vi "sublijnvolgen.vi"(11 "Array":i32[](array[numeric])) -> (3 "Numeric 2":i32)   [LabVIEW 2019]
uses:
  <vilib>/myRIO/Instrument Drivers/Onboard IO/AO/typedefs/AO Reference.ctl
  <vilib>/myRIO/Common/Instrument Driver Framework/Utilities/typedefs/myRIO Generic Hardware Reference.ctl
  <vilib>/myRIO/Common/Instrument Driver Framework/Utilities/typedefs/Hardware Version Enum.ctl
  <vilib>/myRIO/Common/Instrument Driver Framework/Utilities/typedefs/myRIO v1.0 Reference.ctl
  <vilib>/myRIO/Common/Instrument Driver Framework/Utilities/typedefs/Generic FPGA Reference.ctl
  <vilib>/myRIO/Common/Instrument Driver Framework/myRIO v1.0/AO/typedefs/AO Channels List.ctl
  <vilib>/myRIO/Common/Instrument Driver Framework/myRIO v1.0/AO/typedefs/AO Channels Enum.ctl
  <vilib>/myRIO/Common/Instrument Driver Framework/Utilities/typedefs/Analog Scaling Constants List.ctl
  <vilib>/myRIO/Common/Instrument Driver Framework/Utilities/typedefs/Analog Scaling Constants.ctl
  <vilib>/userDefined/High Color/nirio_resource_hc.ctl
  <vilib>/myRIO/Common/Instrument Driver Framework/Utilities/vis/Is FPGA Ref Available.vi
  <vilib>/myRIO/Common/Instrument Driver Framework/myRIO v1.0/AO/vis/myRIO v1.1 Open AO.vi
  <vilib>/myRIO/Instrument Drivers/Onboard IO/AO/vis/Write.vi
  <vilib>/myRIO/Common/Instrument Driver Framework/Utilities/vis/Validate Channels.vi
  <vilib>/myRIO/Common/Instrument Driver Framework/myRIO v1.0/AO/vis/myRIO v1.0 Reserve AO.vi
  <vilib>/myRIO/Common/Instrument Driver Framework/myRIO v1.0/AO/vis/myRIO v1.0 Build MUX Configuration AO.vi
  <vilib>/myRIO/Common/Instrument Driver Framework/myRIO v1.0/Resource Manager/vis/myRIO v1.0 Reserve Channel List.vi
  <vilib>/myRIO/Common/Instrument Driver Framework/myRIO v1.0/Resource Manager/vis/myRIO v1.0 Reserve Channel.vi
  <vilib>/myRIO/Common/Instrument Driver Framework/myRIO v1.0/Resource Manager/vis/myRIO v1.0 Unreserve Channel.vi
  <vilib>/myRIO/Common/Instrument Driver Framework/myRIO v1.0/Resource Manager/vis/myRIO v1.0 Build Mutex Name.vi
  <vilib>/Utility/VariantDataType/GetNumericInfo.vi
  <vilib>/Utility/error.llb/Error Cluster From Error Code.vi
  <vilib>/myRIO/Common/Instrument Driver Framework/myRIO v1.0/myRIO v1.1 Open.vi
  <vilib>/myRIO/Common/Instrument Driver Framework/myRIO v1.0/AO/vis/myRIO v1.0 Get Scaling Constants AO.vi
  <vilib>/myRIO/Common/Instrument Driver Framework/Utilities/vis/IO Manager.vi
  <vilib>/myRIO/Common/Instrument Driver Framework/Utilities/vis/Configuration Manager.vi
  <vilib>/myRIO/Common/Instrument Driver Framework/myRIO v1.0/myRIO v1.0 Close.vi
  <vilib>/myRIO/Common/Instrument Driver Framework/myRIO v1.0/AO/vis/myRIO v1.0 Write AO.vi
  <vilib>/myRIO/Express VI/Onboard IO/AO/AO Express VI.xnode
  <vilib>/myRIO/Instrument Drivers/Onboard IO/AO/vis/myRIO AO Open.xnode
  <vilib>/myRIO/Instrument Drivers/Onboard IO/AO/AO.lvlib
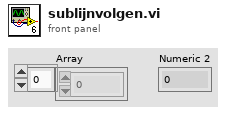
[diagram p1: front panel]
types:
  T1 = typedef "AO.lvlib/AO Reference.ctl" = cluster{"myRIO Reference":T2, "AO Channel List":T6, "AO Scaling Constant List":T8}
  T2 = typedef "myRIO Generic Hardware Reference.ctl" = cluster{"myRIO Model":T3, "myRIO Hardware Reference":T4}
  T3 = typedef "Hardware Version Enum.ctl" = enum16{"Unknown", "myRIO-1900", "myRIO-1950", "roboRIO", "NI ELVIS RIO CM", "ELVIS III"}
  T4 = typedef "myRIO v1.0 Reference.ctl" = cluster{"Generic FPGA Reference":T5, "Allow multiple opens":bool}
  T5 = typedef "Generic FPGA Reference.ctl" = refnum<k20>
  T6 = typedef "AO Channels List.ctl" = T7[]
  T7 = typedef "AO Channels Enum.ctl" = enum16{"Not Connected", "AudioOut/Left", "AudioOut/Right", "C/AO0", "C/AO1", "A/AO0", "A/AO1", "B/AO0", "B/AO1"}
  T8 = typedef "Analog Scaling Constants List.ctl" = T9[]
  T9 = typedef "Analog Scaling Constants.ctl" = cluster{"LSB Weight (Volts)":dbl, "Offset (Volts)":dbl, "Signed?":bool}
  T10 = typedef "nirio_resource_hc.ctl" = tag
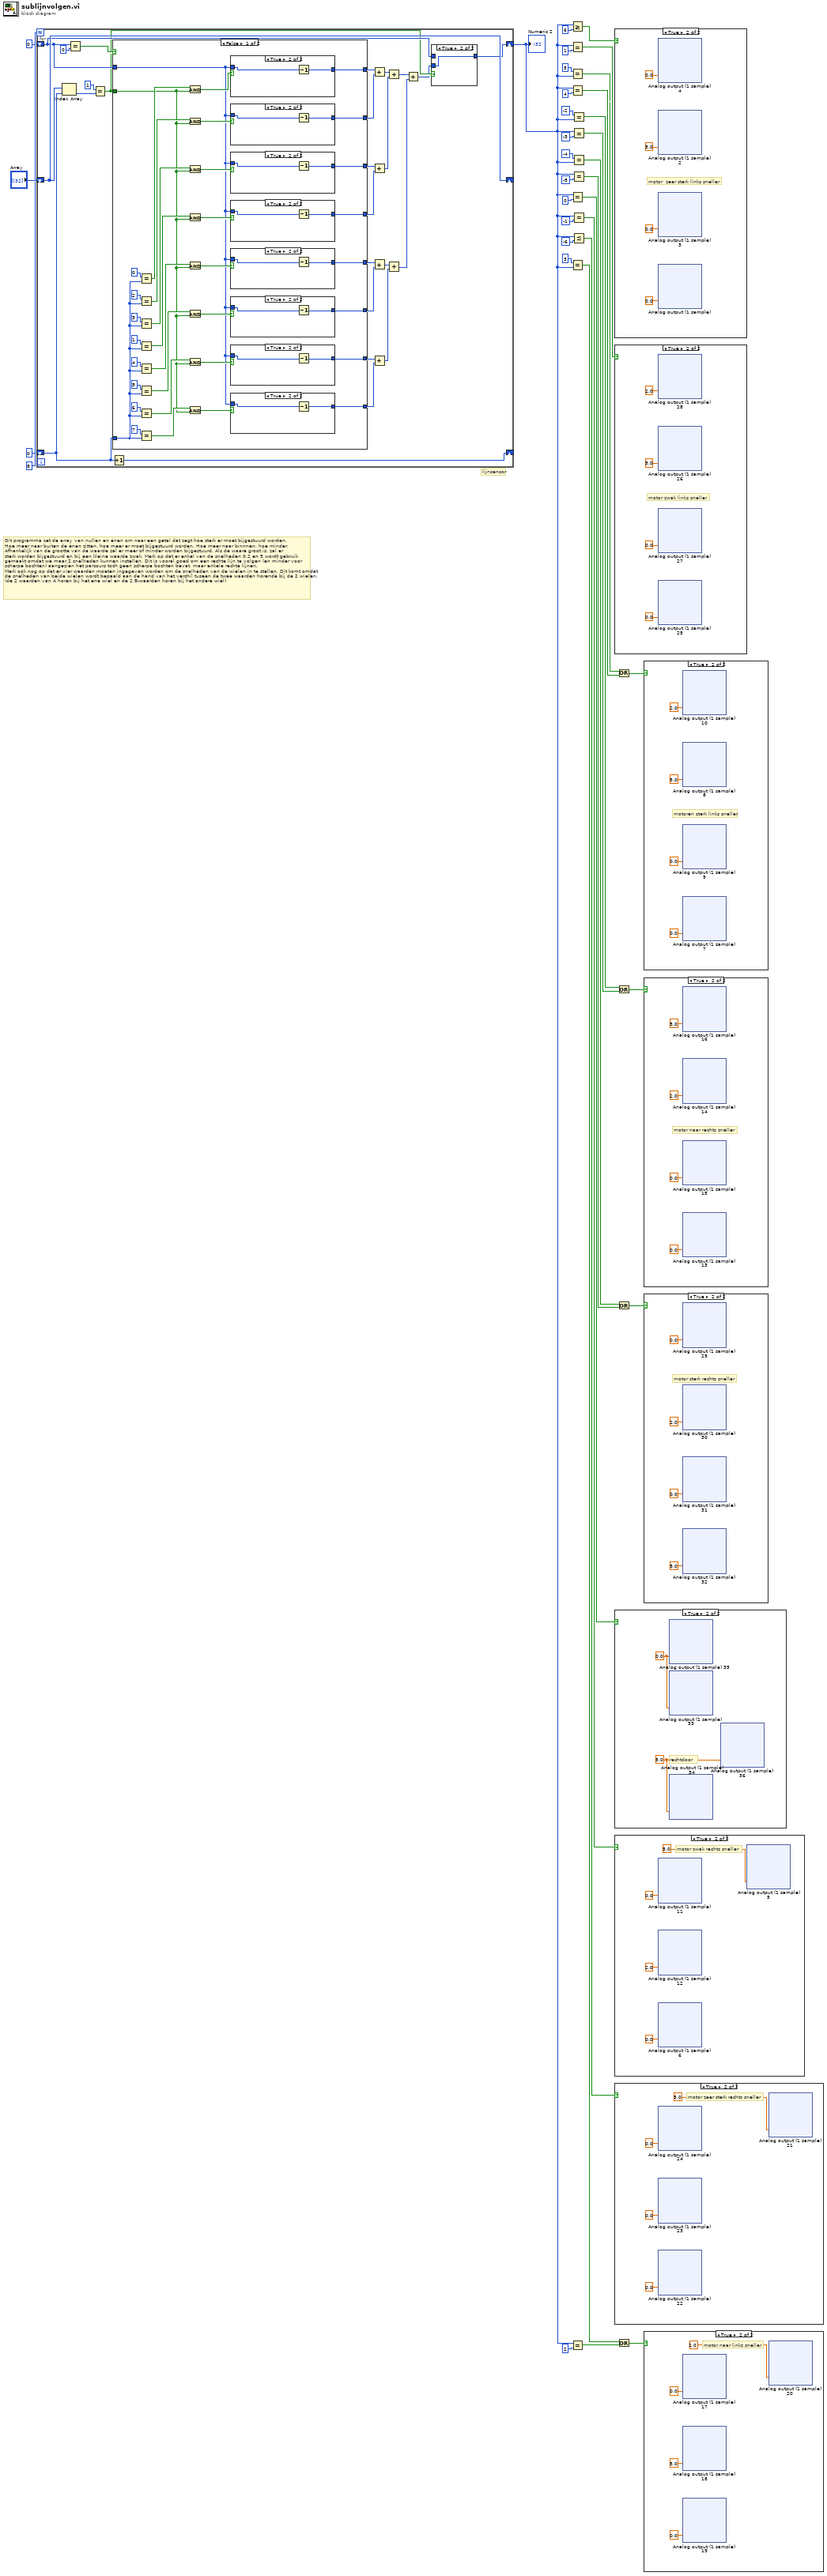
[diagram p0: block diagram]
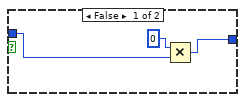
[diagram p12: hidden frame]
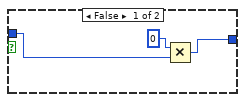
[diagram p13: hidden frame]
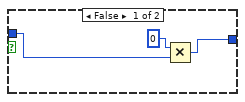
[diagram p14: hidden frame]
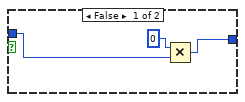
[diagram p15: hidden frame]
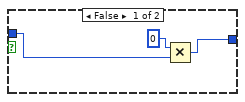
[diagram p16: hidden frame]
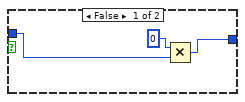
[diagram p17: hidden frame]
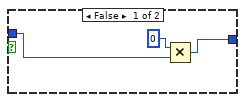
[diagram p18: hidden frame]
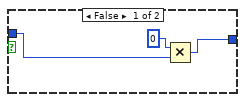
[diagram p19: hidden frame]
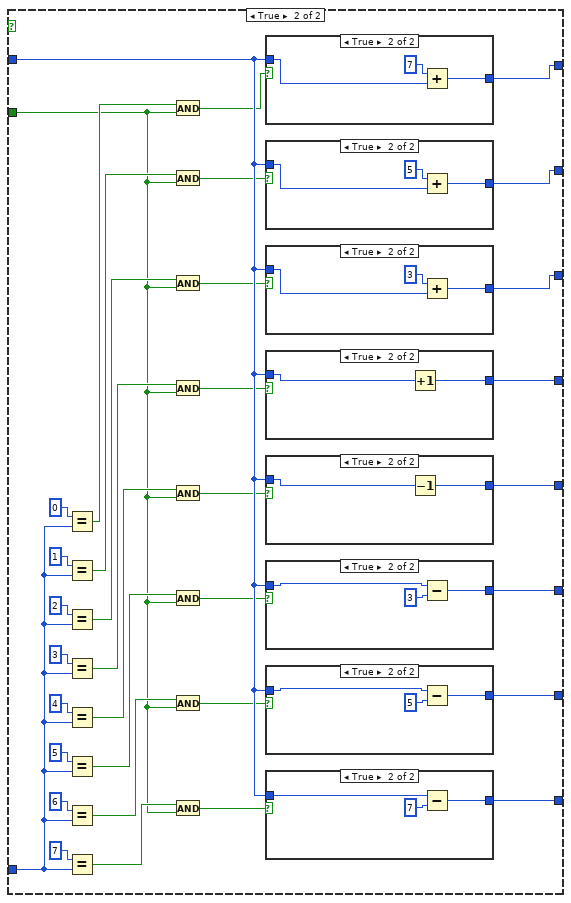
[diagram p20: hidden frame]
diagram:
  # "Dit programma zet de array van nullen en énen om naar een getal dat zegt hoe sterk er moet bijgestuurd worden. \nHoe meer naar buiten de énen zitten, hoe meer er moet bijgestuurd worden. Hoe meer naar binnnen, hoe minder.\nAfhankelijk van de grootte van de waarde zal er meer of minder worden bijgestuurd. Als de waare groot is, zal er \nsterk worden bijgestuurd en bij een kleine waarde zwak. Merk op dat er enkel van de snelheden 0,2 en 5 wordt gebruik\ngemaakt omdat we maar 2 snelheden kunnen instellen. Dit is vooral goed om een rechte lijn te volgen (en minder voor\nscherpe bochten) aangezien het parcours toch geen scherpe bochten bevat, maar enkele rechte lijnen.\nMerk ook nog op dat er vier waarden moeten ingegeven worden om de snelheden van de wielen in te stellen. Dit komt omdat \nde snelheden van beide wielen wordt bepaald aan de hand van het verchil tuseen de twee waarden horende bij de 2 wielen. \n(de 2 waarden van A horen bij het ene wiel en de 2 B-waarden horen bij het andere wiel)"
  # "lijnsensor"
  n1 = for {
    N: 8 -> [_]
    shift-right: [w46] -> _
    shift-left: 0 -> [w60]
    shift-right: [w38] -> w35
    shift-left: 0 -> [w39]
    shift-right: [w51] -> _
    shift-left: "Array" -> [w51]
    n2 = Index Array(array=w51, index=w60) -> (element=w50:i32)
    n3 = Equal?(x=w39, y=0) -> (x = y?=w47:bool)
    n4 = Equal?(x=1, y=w50) -> (x = y?=w37:bool)
    n5 = Increment(x=w60) -> (x+1=w46:i32)
    n6 = case shown="False" w47 {
      tunnel: w60 -> [w70 w156]
      tunnel: [w64 w155] -> w59
      tunnel: [w71 w154] -> w58
      tunnel: [w72 w153] -> w57
      tunnel: [w73 w152] -> w56
      tunnel: w39 -> [w63 w151]
      tunnel: w37 -> [w69 w142]
      tunnel: [w67 w141] -> w45
      tunnel: [w68 w140] -> w44
      tunnel: [w65 w139] -> w42
      tunnel: [w66 w138] -> w41
      frame False {
        n7 = Equal?(x=0, y=w70) -> (x = y?=w90:bool)
        n8 = Equal?(x=2, y=w70) -> (x = y?=w96:bool)
        n9 = Equal?(x=3, y=w70) -> (x = y?=w97:bool)
        n10 = Equal?(x=1, y=w70) -> (x = y?=w82:bool)
        n11 = Equal?(x=4, y=w70) -> (x = y?=w94:bool)
        n12 = Equal?(x=5, y=w70) -> (x = y?=w95:bool)
        n13 = Equal?(x=6, y=w70) -> (x = y?=w93:bool)
        n14 = Equal?(x=7, y=w70) -> (x = y?=w92:bool)
        n15 = And(x=w90, y=w69) -> (x .and. y?=w74:bool)
        n16 = And(x=w96, y=w69) -> (x .and. y?=w76:bool)
        n17 = And(x=w97, y=w69) -> (x .and. y?=w77:bool)
        n18 = And(x=w82, y=w69) -> (x .and. y?=w75:bool)
        n19 = And(x=w94, y=w69) -> (x .and. y?=w78:bool)
        n20 = And(x=w95, y=w69) -> (x .and. y?=w79:bool)
        n21 = And(x=w93, y=w69) -> (x .and. y?=w80:bool)
        n22 = And(x=w92, y=w69) -> (x .and. y?=w81:bool)
        n23 = case shown="True" w74 {
          tunnel: [w99 w102] -> w68
          tunnel: w63 -> [w98 w101]
          frame False {
            n24 = Multiply(x=0, y=w98) -> (x*y=w99:i32)
          }
          frame True {
            n25 = Decrement(x=w101) -> (x-1=w102:i32)
          }
        }
        n26 = case shown="True" w76 {
          tunnel: [w130 w131] -> w67
          tunnel: w63 -> [w129 w132]
          frame False {
            n27 = Multiply(x=0, y=w129) -> (x*y=w130:i32)
          }
          frame True {
            n28 = Decrement(x=w132) -> (x-1=w131:i32)
          }
        }
        n29 = case shown="True" w77 {
          tunnel: [w124 w127] -> w66
          tunnel: w63 -> [w123 w126]
          frame False {
            n30 = Multiply(x=0, y=w123) -> (x*y=w124:i32)
          }
          frame True {
            n31 = Decrement(x=w126) -> (x-1=w127:i32)
          }
        }
        n32 = case shown="True" w75 {
          tunnel: [w134 w137] -> w65
          tunnel: w63 -> [w133 w136]
          frame False {
            n33 = Multiply(x=0, y=w133) -> (x*y=w134:i32)
          }
          frame True {
            n34 = Decrement(x=w136) -> (x-1=w137:i32)
          }
        }
        n35 = case shown="True" w78 {
          tunnel: [w119 w122] -> w64
          tunnel: w63 -> [w118 w121]
          frame False {
            n36 = Multiply(x=0, y=w118) -> (x*y=w119:i32)
          }
          frame True {
            n37 = Decrement(x=w121) -> (x-1=w122:i32)
          }
        }
        n38 = case shown="True" w79 {
          tunnel: [w109 w112] -> w71
          tunnel: w63 -> [w108 w111]
          frame False {
            n39 = Multiply(x=0, y=w108) -> (x*y=w109:i32)
          }
          frame True {
            n40 = Decrement(x=w111) -> (x-1=w112:i32)
          }
        }
        n41 = case shown="True" w80 {
          tunnel: [w114 w117] -> w72
          tunnel: w63 -> [w113 w116]
          frame False {
            n42 = Multiply(x=0, y=w113) -> (x*y=w114:i32)
          }
          frame True {
            n43 = Decrement(x=w116) -> (x-1=w117:i32)
          }
        }
        n44 = case shown="True" w81 {
          tunnel: [w103 w107] -> w73
          tunnel: w63 -> [w104 w106]
          frame False {
            n45 = Multiply(x=0, y=w104) -> (x*y=w103:i32)
          }
          frame True {
            n46 = Decrement(x=w106) -> (x-1=w107:i32)
          }
        }
      }
      frame True {
        n47 = Equal?(x=0, y=w156) -> (x = y?=w165:bool)
        n48 = Equal?(x=1, y=w156) -> (x = y?=w157:bool)
        n49 = Equal?(x=2, y=w156) -> (x = y?=w171:bool)
        n50 = Equal?(x=3, y=w156) -> (x = y?=w172:bool)
        n51 = Equal?(x=4, y=w156) -> (x = y?=w169:bool)
        n52 = Equal?(x=5, y=w156) -> (x = y?=w170:bool)
        n53 = Equal?(x=6, y=w156) -> (x = y?=w168:bool)
        n54 = Equal?(x=7, y=w156) -> (x = y?=w167:bool)
        n55 = And(x=w165, y=w142) -> (x .and. y?=w143:bool)
        n56 = And(x=w157, y=w142) -> (x .and. y?=w144:bool)
        n57 = And(x=w171, y=w142) -> (x .and. y?=w145:bool)
        n58 = And(x=w172, y=w142) -> (x .and. y?=w146:bool)
        n59 = And(x=w169, y=w142) -> (x .and. y?=w147:bool)
        n60 = And(x=w170, y=w142) -> (x .and. y?=w148:bool)
        n61 = And(x=w168, y=w142) -> (x .and. y?=w149:bool)
        n62 = And(x=w167, y=w142) -> (x .and. y?=w150:bool)
        n63 = case shown="True" w143 {
          tunnel: w151 -> [w173 w177]
          tunnel: [w174 w176] -> w140
          frame False {
            n64 = Multiply(x=0, y=w173) -> (x*y=w174:i32)
          }
          frame True {
            n65 = Add(x=7, y=w177) -> (x+y=w176:i32)
          }
        }
        n66 = case shown="True" w144 {
          tunnel: w151 -> [w213 w216]
          tunnel: [w214 w217] -> w141
          frame False {
            n67 = Multiply(x=0, y=w213) -> (x*y=w214:i32)
          }
          frame True {
            n68 = Add(x=5, y=w216) -> (x+y=w217:i32)
          }
        }
        n69 = case shown="True" w145 {
          tunnel: w151 -> [w207 w211]
          tunnel: [w208 w210] -> w138
          frame False {
            n70 = Multiply(x=0, y=w207) -> (x*y=w208:i32)
          }
          frame True {
            n71 = Add(x=3, y=w211) -> (x+y=w210:i32)
          }
        }
        n72 = case shown="True" w146 {
          tunnel: w151 -> [w203 w206]
          tunnel: [w202 w205] -> w139
          frame False {
            n73 = Multiply(x=0, y=w203) -> (x*y=w202:i32)
          }
          frame True {
            n74 = Increment(x=w206) -> (x+1=w205:i32)
          }
        }
        n75 = case shown="True" w147 {
          tunnel: w151 -> [w197 w201]
          tunnel: [w198 w200] -> w155
          frame False {
            n76 = Multiply(x=0, y=w197) -> (x*y=w198:i32)
          }
          frame True {
            n77 = Decrement(x=w201) -> (x-1=w200:i32)
          }
        }
        n78 = case shown="True" w148 {
          tunnel: w151 -> [w186 w188]
          tunnel: [w185 w190] -> w154
          frame False {
            n79 = Multiply(x=0, y=w186) -> (x*y=w185:i32)
          }
          frame True {
            n80 = Subtract(x=w188, y=3) -> (x-y=w190:i32)
          }
        }
        n81 = case shown="True" w149 {
          tunnel: w151 -> [w192 w194]
          tunnel: [w191 w195] -> w153
          frame False {
            n82 = Multiply(x=0, y=w192) -> (x*y=w191:i32)
          }
          frame True {
            n83 = Subtract(x=w194, y=5) -> (x-y=w195:i32)
          }
        }
        n84 = case shown="True" w150 {
          tunnel: w151 -> [w179 w182]
          tunnel: [w180 w183] -> w152
          frame False {
            n85 = Multiply(x=0, y=w179) -> (x*y=w180:i32)
          }
          frame True {
            n86 = Subtract(x=w182, y=7) -> (x-y=w183:i32)
          }
        }
      }
    }
    n87 = Add(x=w44, y=w45) -> (x+y=w43:i32)
    n88 = Add(x=w41, y=w42) -> (x+y=w40:i32)
    n89 = Add(x=w59, y=w58) -> (x+y=w54:i32)
    n90 = Add(x=w57, y=w56) -> (x+y=w55:i32)
    n91 = Add(x=w43, y=w40) -> (x+y=w53:i32)
    n92 = Add(x=w54, y=w55) -> (x+y=w52:i32)
    n93 = Add(x=w53, y=w52) -> (x+y=w36:i32)
    n94 = case shown="True" w37 {
      tunnel: w39 -> [w61 _]
      tunnel: [w61 w62] -> w38
      tunnel: w36 -> [_ w62]
      frame False {
      }
      frame True {
      }
    }
  }
  "Numeric 2" <- w35
  n95 = Greater Or Equal?(x=w35, y=6) -> (x >= y?=w6:bool)
  n96 = Equal?(x=w35, y=1) -> (x = y?=w5:bool)
  n97 = Equal?(x=5, y=w35) -> (x = y?=w11:bool)
  n98 = Equal?(x=w35, y=4) -> (x = y?=w10:bool)
  n99 = Equal?(x=w35, y=0) -> (x = y?=w34:bool)
  n100 = Equal?(x=3, y=w35) -> (x = y?=w15:bool)
  n101 = Equal?(x=w35, y=2) -> (x = y?=w14:bool)
  n102 = Equal?(x=-2, y=w35) -> (x = y?=w21:bool)
  n103 = Equal?(x=w35, y=-3) -> (x = y?=w20:bool)
  n104 = Equal?(x=-4, y=w35) -> (x = y?=w25:bool)
  n105 = Equal?(x=w35, y=-5) -> (x = y?=w24:bool)
  n106 = Equal?(x=w35, y=-1) -> (x = y?=w27:bool)
  n107 = Less Or Equal?(x=w35, y=-6) -> (x <= y?=w29:bool)
  n108 = case shown="True" w6 {
    frame False {
    }
    frame True {
      # "motor  zeer sterk links sneller"
      n109 = xnode "Analog output (1 sample) 4"("A/AO0 (Pin 2)"=0.0) -> ()  [unwired: 1 in, 1 out]
      n110 = xnode "Analog output (1 sample) 2"("B/AO0 (Pin 2)"=5.0) -> ()  [unwired: 1 in, 1 out]
      n111 = xnode "Analog output (1 sample) 3"("A/AO1 (Pin 4)"=0.0) -> ()  [unwired: 1 in, 1 out]
      n112 = xnode "Analog output (1 sample)"("B/AO1 (Pin 4)"=0.0) -> ()  [unwired: 1 in, 1 out]
    }
  }
  n113 = case shown="True" w5 {
    frame False {
    }
    frame True {
      # "motor zwak links sneller"
      n114 = xnode "Analog output (1 sample) 28"("A/AO0 (Pin 2)"=2.0) -> ()  [unwired: 1 in, 1 out]
      n115 = xnode "Analog output (1 sample) 26"("B/AO0 (Pin 2)"=5.0) -> ()  [unwired: 1 in, 1 out]
      n116 = xnode "Analog output (1 sample) 27"("A/AO1 (Pin 4)"=0.0) -> ()  [unwired: 1 in, 1 out]
      n117 = xnode "Analog output (1 sample) 25"("B/AO1 (Pin 4)"=0.0) -> ()  [unwired: 1 in, 1 out]
    }
  }
  n118 = case shown="True" w34 {
    frame False {
    }
    frame True {
      w524 = 0.0
      w523 = 5.0
      # "rechtdoor"
      n119 = xnode "Analog output (1 sample) 35"("A/AO1 (Pin 4)"=w524) -> ()  [unwired: 1 in, 1 out]
      n120 = xnode "Analog output (1 sample) 33"("B/AO1 (Pin 4)"=w524) -> ()  [unwired: 1 in, 1 out]
      n121 = xnode "Analog output (1 sample) 34"("B/AO0 (Pin 2)"=w523) -> ()  [unwired: 1 in, 1 out]
      n122 = xnode "Analog output (1 sample) 36"("A/AO0 (Pin 2)"=w523) -> ()  [unwired: 1 in, 1 out]
    }
  }
  n123 = case shown="True" w27 {
    frame False {
    }
    frame True {
      # "motor zwak rechts sneller"
      n124 = xnode "Analog output (1 sample) 11"("B/AO1 (Pin 4)"=0.0) -> ()  [unwired: 1 in, 1 out]
      n125 = xnode "Analog output (1 sample) 12"("B/AO0 (Pin 2)"=2.0) -> ()  [unwired: 1 in, 1 out]
      n126 = xnode "Analog output (1 sample) 6"("A/AO1 (Pin 4)"=0.0) -> ()  [unwired: 1 in, 1 out]
      n127 = xnode "Analog output (1 sample) 5"("A/AO0 (Pin 2)"=5.0) -> ()  [unwired: 1 in, 1 out]
    }
  }
  n128 = case shown="True" w29 {
    frame False {
    }
    frame True {
      # "motor zeer sterk rechts sneller"
      n129 = xnode "Analog output (1 sample) 24"("B/AO1 (Pin 4)"=0.0) -> ()  [unwired: 1 in, 1 out]
      n130 = xnode "Analog output (1 sample) 23"("B/AO0 (Pin 2)"=0.0) -> ()  [unwired: 1 in, 1 out]
      n131 = xnode "Analog output (1 sample) 22"("A/AO1 (Pin 4)"=0.0) -> ()  [unwired: 1 in, 1 out]
      n132 = xnode "Analog output (1 sample) 21"("A/AO0 (Pin 2)"=5.0) -> ()  [unwired: 1 in, 1 out]
    }
  }
  n133 = Or(x=w11, y=w10) -> (x .or. y?=w9:bool)
  n134 = Or(x=w21, y=w20) -> (x .or. y?=w28:bool)
  n135 = Or(x=w25, y=w24) -> (x .or. y?=w31:bool)
  n136 = Or(x=w15, y=w14) -> (x .or. y?=w17:bool)
  n137 = case shown="True" w9 {
    frame False {
    }
    frame True {
      # "motoren sterk links sneller"
      n138 = xnode "Analog output (1 sample) 10"("A/AO0 (Pin 2)"=2.0) -> ()  [unwired: 1 in, 1 out]
      n139 = xnode "Analog output (1 sample) 8"("B/AO0 (Pin 2)"=5.0) -> ()  [unwired: 1 in, 1 out]
      n140 = xnode "Analog output (1 sample) 9"("A/AO1 (Pin 4)"=0.0) -> ()  [unwired: 1 in, 1 out]
      n141 = xnode "Analog output (1 sample) 7"("B/AO1 (Pin 4)"=0.0) -> ()  [unwired: 1 in, 1 out]
    }
  }
  n142 = case shown="True" w28 {
    frame False {
    }
    frame True {
      # "motor naar rechts sneller"
      n143 = xnode "Analog output (1 sample) 16"("A/AO0 (Pin 2)"=5.0) -> ()  [unwired: 1 in, 1 out]
      n144 = xnode "Analog output (1 sample) 14"("B/AO0 (Pin 2)"=2.0) -> ()  [unwired: 1 in, 1 out]
      n145 = xnode "Analog output (1 sample) 15"("A/AO1 (Pin 4)"=0.0) -> ()  [unwired: 1 in, 1 out]
      n146 = xnode "Analog output (1 sample) 13"("B/AO1 (Pin 4)"=0.0) -> ()  [unwired: 1 in, 1 out]
    }
  }
  n147 = case shown="True" w31 {
    frame False {
    }
    frame True {
      # "motor sterk rechts sneller"
      n148 = xnode "Analog output (1 sample) 29"("B/AO1 (Pin 4)"=0.0) -> ()  [unwired: 1 in, 1 out]
      n149 = xnode "Analog output (1 sample) 30"("B/AO0 (Pin 2)"=2.0) -> ()  [unwired: 1 in, 1 out]
      n150 = xnode "Analog output (1 sample) 31"("A/AO1 (Pin 4)"=0.0) -> ()  [unwired: 1 in, 1 out]
      n151 = xnode "Analog output (1 sample) 32"("A/AO0 (Pin 2)"=5.0) -> ()  [unwired: 1 in, 1 out]
    }
  }
  n152 = case shown="True" w17 {
    frame False {
    }
    frame True {
      # "motor naar links sneller"
      n153 = xnode "Analog output (1 sample) 17"("B/AO1 (Pin 4)"=0.0) -> ()  [unwired: 1 in, 1 out]
      n154 = xnode "Analog output (1 sample) 18"("B/AO0 (Pin 2)"=5.0) -> ()  [unwired: 1 in, 1 out]
      n155 = xnode "Analog output (1 sample) 19"("A/AO1 (Pin 4)"=0.0) -> ()  [unwired: 1 in, 1 out]
      n156 = xnode "Analog output (1 sample) 20"("A/AO0 (Pin 2)"=2.0) -> ()  [unwired: 1 in, 1 out]
    }
  }
